vi "GOOP_GetCustomClassTemplates.vi"(10 "ClassType":string) -> (3 "CustomTemplates":path[](array[path]))   [LabVIEW 2020]
uses:
  <vilib>/Utility/config.llb/Read Key (Path).vi
  <vilib>/Utility/config.llb/NI_LVConfig.lvlib
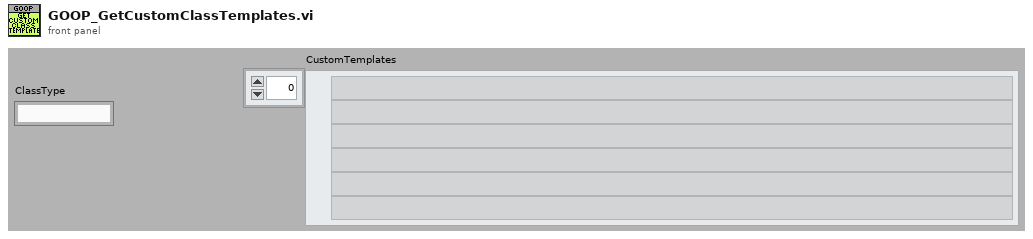
[diagram p1: front panel]
types:
  T1 = typedef "NI_LVConfig.lvlib/Config Data RefNum.ctl" = refnum<k1>
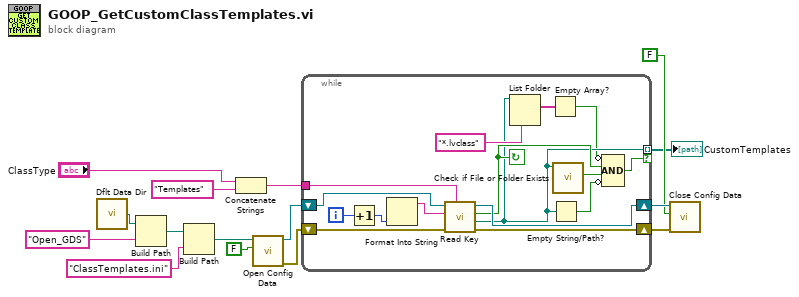
[diagram p0: block diagram]
diagram:
  n1 = call <vilib>:"Dflt Data Dir.vi"() -> ("App:Default Data Directory"=w15:path)
  n2 = Build Path(base path=w15, name or relative path="Open_GDS") -> (appended path=w13:path)
  n3 = Build Path(base path=w13, name or relative path="ClassTemplates.ini") -> (appended path=w2:path)
  n4 = Concatenate Strings("ClassType", "Templates" ("string")) -> (w3:string)
  n5 = call <vilib>:"Open Config Data.vi"("create file if necessary (T)"=FALSE, "configuration file path"=w2) -> ("error out"=w10:errorcluster, "refnum"=w11:T1)  [unwired: 7 in, 1 out]
  n6 = while {
    tunnel: [w17] -> w1 mode=indexing if=w20
    tunnel: w3 -> [w27]
    shift-right: [w29] -> w8
    shift-left: w11 -> [w31]
    shift-right: [w28] -> w7
    shift-left: w10 -> [w30]
    i -> [w26]
    stop <- w23 continue-if-true
    n7 = Increment(x=w26) -> (x+1=w25:i32)
    n8 = Format Into String(w25) -> (resulting string=w24:string)  [unwired: 3 in, 1 out]
    n9 = call-poly <vilib>:"Read Key.vi"("section"=w27, "error in (no error)"=w30, "key"=w24, "refnum"=w31) -> ("error out"=w28:errorcluster, "value"=w17:path, "found?"=w23:bool, "refnum out"=w29:T1)  [unwired: 4 in]
    n10 = List Folder(path=w17, pattern="*.lvclass") -> (filenames=w18:string[])  [unwired: 2 in, 3 out]
    n11 = Empty Array?(array=w18) -> (empty?=w16:bool)
    n12 = Empty String/Path?(string/path=w17) -> (empty?=w21:bool)
    n13 = call <vilib>:"Check if File or Folder Exists.vi"("path"=w17) -> ("file or folder exists?"=w22:bool)  [unwired: 8 in, 2 out]
    n14 = Compound Arithmetic op=AND(invert w16, w23, w22, invert w21) -> (w20:bool)
  }
  "CustomTemplates" <- w1
  n15 = call <vilib>:"Close Config Data.vi"("error in (no error)"=w7, "write file if changed (T)"=FALSE ("create file if necessary (T)"), "refnum"=w8) -> ()  [unwired: 7 in, 2 out]
